vi "Configure Voltage Offset.vi"(0 "VISA resource name":refnum<visa-resource-name>, 1 "Voltage Offset Slew Rate (9.9E+37 V)":dbl=9.9e+37 format="%#.4g", 2 "Voltage Offset Slew Mode (0: Fix)":u16(ring) items=["Fixed", "Step", "Pulse", "List"], 5 "Voltage Offset (0 V)":dbl format="%#.4g", 7 "Voltage Offset Mode (0: Fix)":u16(ring) items=["Fixed", "Step", "Pulse", "List"], 11 "error in (no error)":errorcluster, 12 "Triggered Voltage Offset (0 V)":dbl format="%#.4g", 13 "Triggered Voltage Offset Slew Rate (9.9E+37 V)":dbl=9.9e+37 format="%#.4g") -> (4 "VISA resource name out":refnum<visa-resource-name>, 15 "error out":errorcluster)   [LabVIEW 2020, in "Agilent 681x Series.lvlib"]
doc: "Configures the voltage offset settings of the instrument."
uses:
  <instrlib>/Agilent 681x Series/Agilent 681x Series.lvlib
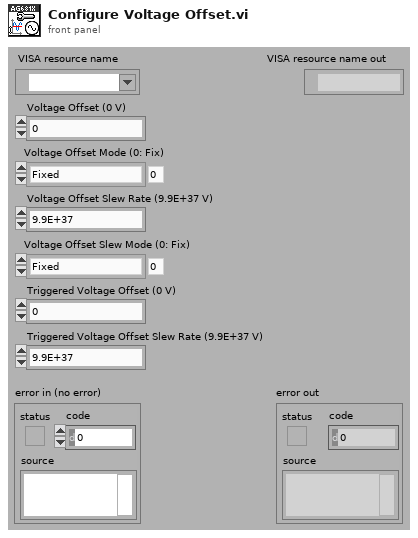
[diagram p1: front panel]
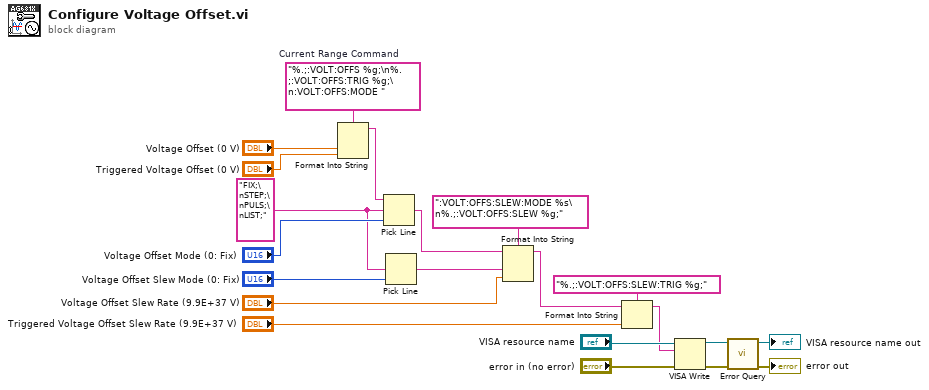
[diagram p0: block diagram]
diagram:
  w9 = "FIX;\nSTEP;\nPULS;\nLIST;" ("multi-line string")
  w17 = "%.;:VOLT:OFFS %g;\n%.;:VOLT:OFFS:TRIG %g;\n:VOLT:OFFS:MODE "  # Current Range Command
  n1 = Format Into String(format string=w17, "Voltage Offset (0 V)", "Triggered Voltage Offset (0 V)") -> (resulting string=w14:string)  [unwired: 2 in, 1 out]
  n2 = Pick Line(string ("")=w14, multi-line string=w9, line index="Voltage Offset Mode (0: Fix)") -> (output string=w3:string)
  n3 = Pick Line(multi-line string=w9, line index="Voltage Offset Slew Mode (0: Fix)") -> (output string=w10:string)  [unwired: 1 in]
  n4 = Format Into String(format string=":VOLT:OFFS:SLEW:MODE %s\n%.;:VOLT:OFFS:SLEW %g;", initial string=w3, w10, "Voltage Offset Slew Rate (9.9E+37 V)") -> (resulting string=w7:string)  [unwired: 1 in, 1 out]
  n5 = Format Into String(format string="%.;:VOLT:OFFS:SLEW:TRIG %g;", initial string=w7, "Triggered Voltage Offset Slew Rate (9.9E+37 V)") -> (resulting string=w5:string)  [unwired: 1 in, 1 out]
  n6 = VISA Write(VISA resource name="VISA resource name", write buffer=w5, error in (no error)="error in (no error)") -> (VISA resource name out=w19:refnum<visa-resource-name>, error out=w18:errorcluster)  [unwired: 1 out]
  n7 = call <instrlib>:"Error Query.vi"("error in (no error)"=w18, "VISA resource name"=w19) -> ("error out"=→"error out":errorcluster, "VISA resource name out"=→"VISA resource name out":refnum<visa-resource-name>)  [unwired: 6 in, 2 out]
